vi "Generate 1kHz const signal for every channel  (SubVI).vi"(11 "single data for evry channel":dbl[](array[numeric])) -> (3 "Buffor":dbl[](array[numeric]))   [LabVIEW 2009, in "MicroDAQ.lvlib" / "Analog output.lvclass"]
uses:
  <instrlib>/MicroDAQ/Channel/Analog Output/Analog output.lvclass
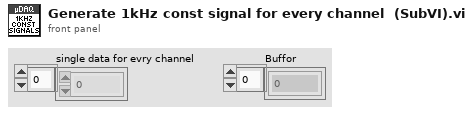
[diagram p1: front panel]
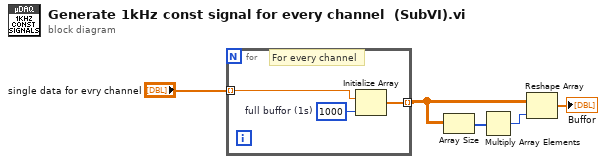
[diagram p0: block diagram]
diagram:
  n1 = for {
    tunnel: "single data for evry channel" -> [w7] mode=indexing
    tunnel: [w6] -> w5 mode=indexing
    w8 = 1000  # full buffor (1s)
    # "For every channel"
    n2 = Initialize Array(w7, w8) -> (w6:dbl[])
  }
  n3 = Array Size(array=w5) -> (size(s)=w3:i32[])
  n4 = Multiply Array Elements(1:w3) -> (0:w4:i32)
  n5 = Reshape Array(w5, w4) -> (→"Buffor":dbl[])
